vi "Linear_Distance.vi"(10 "Axle Radius":dbl=0.0045 format="%#_13g", 11 "Number Of Rotations":dbl) -> (3 "Linear Distance":dbl)   [LabVIEW 2018]
doc: "This VI calculates current linear distance by multiplying current number of rotations by circumference of encoder shaft.\n\nInputs:\nNumber of rotations;\nAxle Radius.\n\nOutputs:\nLinear distance."
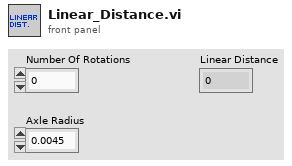
[diagram p1: front panel]
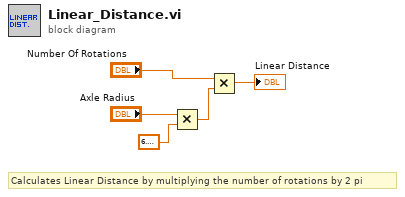
[diagram p0: block diagram]
diagram:
  # "Calculates Linear Distance by multiplying the number of rotations by 2 pi"
  n1 = Multiply(x="Axle Radius", y=6.283185307179586) -> (x*y=w5:dbl)
  n2 = Multiply(x="Number Of Rotations", y=w5) -> (x*y=→"Linear Distance":dbl)
